vi "Read Error Queue.vi"(8 "error in (no error)":errorcluster, 11 "Performanced XNET CAN Signal Logger in":refnum<class "Performanced XNET CAN Logger.lvclass">) -> (0 "error out":errorcluster, 2 "Error Queue":refnum<queue>, 3 "Performanced XNET CAN Signal Logger out":refnum<class "Performanced XNET CAN Logger.lvclass">)   [LabVIEW 2021, in "Performanced XNET CAN Logger.lvlib" / "Performanced XNET CAN Logger.lvclass"]
uses:
  Performanced XNET CAN Logger.lvclass
  Performanced XNET CAN Logger.lvclass/Performanced XNET CAN Logger.ctl
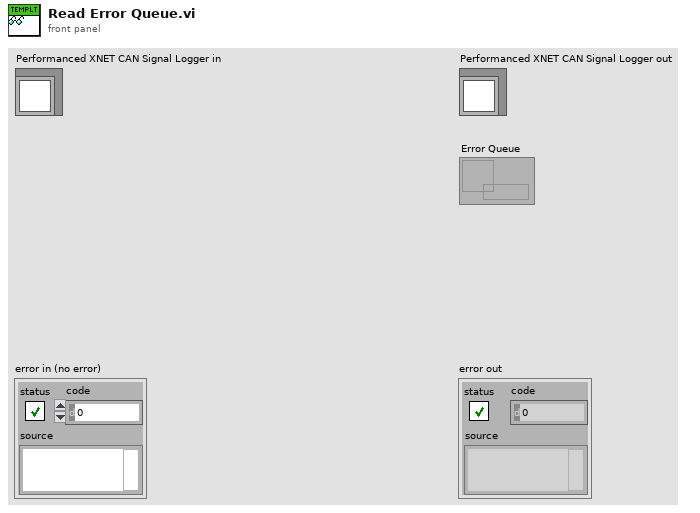
[diagram p1: front panel]
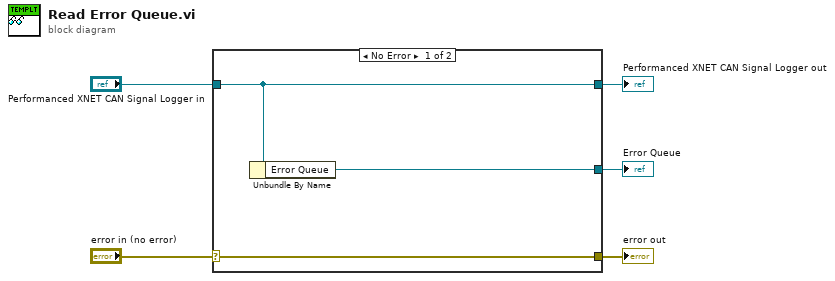
[diagram p0: block diagram]
diagram:
  n1 = case shown="No Error" "error in (no error)" {
    selector: "error in (no error)" -> [w8 w9]
    tunnel: [w8 w9] -> w4
    tunnel: [w7 w10] -> w2
    tunnel: "Performanced XNET CAN Signal Logger in" -> [w7 w10]
    tunnel: [w6 _] -> w1
    frame No Error {
      n2 = Unbundle By Name(w7) -> ("Error Queue"=w6:refnum<queue>)
    }
    frame Error {
    }
  }
  "error out" <- w4
  "Performanced XNET CAN Signal Logger out" <- w2
  "Error Queue" <- w1
